vi "CleanDependencies.vi"(8 "error in (no error)":errorcluster, 10 "Dependency":refnum<class "SMO.lvclass">, 11 "SMO in":refnum<class "SMO.lvclass">) -> (0 "error out":errorcluster, 3 "SMO out":refnum<class "SMO.lvclass">, 4 "Removed":bool)   [LabVIEW 2021, in "smo.lvlib" / "SMO.lvclass"]
uses:
  SMO.lvclass
  SMO.lvclass/SMO.ctl
  GetVariant(Attr).vi
  ReftoDVR--SMO.vi
  Support/Attribute.Dependencies/Attribute.Dependencies.lvclass
  C:/Repositories/SMO/src/Support/Attribute/Attribute.lvclass
  Support/Attribute.Dependencies/Get GUIDs.vi
  C:/Repositories/SMO/src/Support/Attribute.Dependencies/Attribute.Dependencies.lvclass
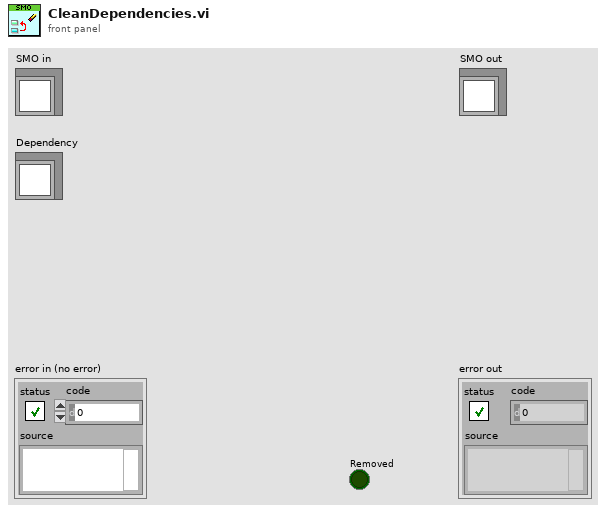
[diagram p1: front panel]
types:
  T1 = typedef "smo.lvlib/Attribute.Dependencies.lvclass/DependencyAttr--Cluster.ctl" = cluster{"Name":string, "GUID":string, "owned":bool, "shared":bool, "Level":string, "SMO":refnum<class "SMO.lvclass">}
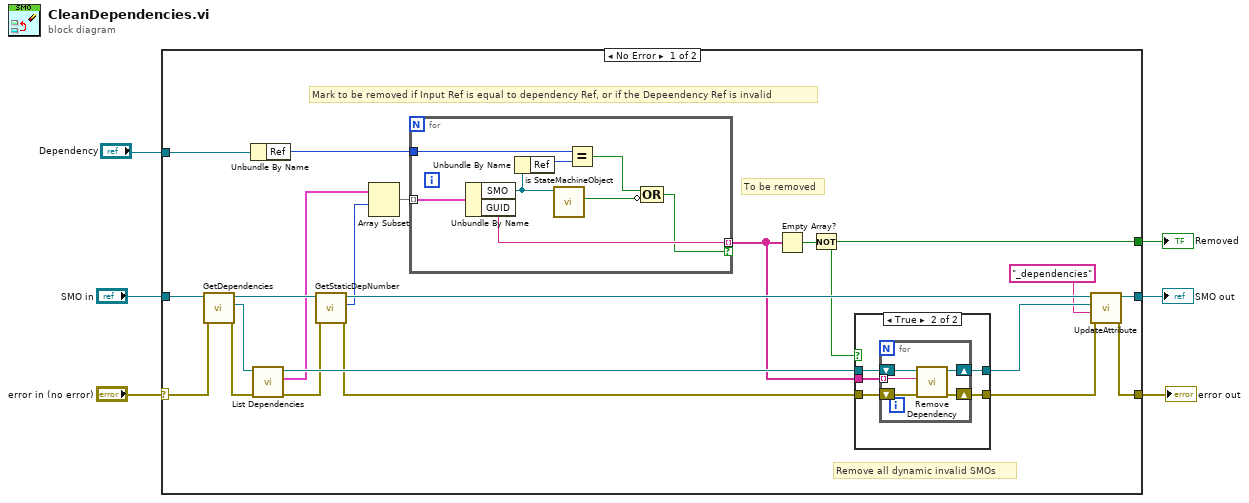
[diagram p0: block diagram]
diagram:
  n1 = case shown="No Error" "error in (no error)" {
    selector: "error in (no error)" -> [w7 w49]
    tunnel: "Dependency" -> [w28 _]
    tunnel: "SMO in" -> [w25 w50]
    tunnel: [w20 w50] -> w4
    tunnel: [w18 w49] -> w3
    tunnel: [w15 _] -> w2
    frame No Error {
      # "Mark to be removed if Input Ref is equal to dependency Ref, or if the Depeendency Ref is invalid"
      # "To be removed"
      # "Remove all dynamic invalid SMOs"
      n2 = call "GetDependencies.vi"("error in (no error)"=w7, "SMO in"=w25) -> ("error out"=w24:errorcluster, "Dependencies"=w26:refnum<class "Attribute.Dependencies.lvclass">, "SMO out"=w23:refnum<class "SMO.lvclass">)  [unwired: 7 in]
      n3 = Unbundle By Name(w28) -> ("Ref"=w27:u32)
      n4 = call "List Dependencies.vi"("error in (no error)"=w24, "Attribute.Dependencies in"=w26) -> ("error out"=w13:errorcluster, "Dependencies"=w10:T1[], "Attribute.Dependencies out"=w16:refnum<class "Attribute.Dependencies.lvclass">)  [unwired: 7 in]
      n5 = call "GetStaticDepNumber.vi"("error in (no error)"=w13, "SMO in"=w23) -> ("error out"=w12:errorcluster, "Nb of Static Dependencies"=w11:u32, "SMO out"=w21:refnum<class "SMO.lvclass">)  [unwired: 7 in]
      n6 = Array Subset(array=w10, index=w11) -> (w9:T1[])  [unwired: 1 in]
      n7 = for {
        tunnel: [w43] -> w14 mode=indexing if=w41
        tunnel: w27 -> [w47]
        tunnel: w9 -> [w44] mode=indexing
        n8 = Unbundle By Name(w44) -> ("SMO"=w48:refnum<class "SMO.lvclass">, "GUID"=w43:string)
        n9 = Unbundle By Name(w48) -> ("Ref"=w46:u32)
        n10 = call "is StateMachineObject.vi"("SMO"=w48) -> ("is SMO?"=w42:bool)  [unwired: 8 in, 2 out]
        n11 = Equal?(x=w47, y=w46) -> (x = y?=w45:bool)
        n12 = Compound Arithmetic op=OR(w45, invert w42) -> (w41:bool)
      }
      n13 = Empty Array?(array=w14) -> (empty?=w22:bool)
      n14 = Not(x=w22) -> (.not. x?=w15:bool)
      n15 = case shown="True" w15 {
        tunnel: [w30 w35] -> w19
        tunnel: [w29 w34] -> w17
        tunnel: w12 -> [w29 w33]
        tunnel: w16 -> [w30 w32]
        tunnel: w14 -> [_ w31]
        frame False {
        }
        frame True {
          n16 = for {
            shift-right: [w40] -> w35
            shift-left: w32 -> [w38]
            shift-right: [w39] -> w34
            shift-left: w33 -> [w37]
            tunnel: w31 -> [w36] mode=indexing
            n17 = call "Remove Dependency.vi"("error in (no error)"=w37, "GUID"=w36, "Attribute.Dependencies in"=w38) -> ("error out"=w39:errorcluster, "Attribute.Dependencies out"=w40:refnum<class "Attribute.Dependencies.lvclass">)  [unwired: 7 in]
          }
        }
      }
      n18 = call "UpdateAttribute.vi"("error in (no error)"=w17, "Attribute Name"="_dependencies", "Attribute"=w19, "SMO in"=w21) -> ("error out"=w18:errorcluster, "SMO in"=w20:refnum<class "SMO.lvclass">)  [unwired: 5 in, 1 out]
    }
    frame Error {
    }
  }
  "error out" <- w3
  "SMO out" <- w4
  "Removed" <- w2
